vi "Read Return Address.vi"(11 "PreAddressedMsg in":refnum<class "PreAddressedMsg.lvclass">) -> (1 "Return Priority (Normal)":T1=enum."Normal", 2 "Return Address":refnum<class "Message Enqueuer.lvclass">)   [LabVIEW 2017, in "AbstractMessages.lvlib" / "PreAddressedMsg.lvclass"]
doc: "<License>\nCopyright © 2017 Composed Systems, LLC | All rights reserved\nwww.composed.io\n\nAuthor: Ethan Stern <ethan.stern@composed.io>\n\nThis software is provided \"AS IS\" WITHOUT WARRANTIES, either express or implied, AND IS FOR EDUCATIONAL PURPOSES ONLY.\n</License>"
uses:
  PreAddressedMsg.lvclass
  <vilib>/ActorFramework/Message Enqueuer/Message Enqueuer.lvclass
  <vilib>/ActorFramework/Message Enqueuer/Message Priority.ctl
  PreAddressedMsg.lvclass/PreAddressedMsg.ctl
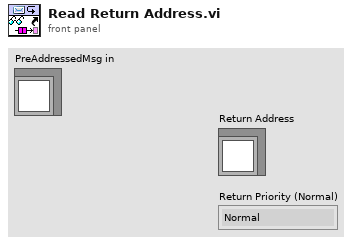
[diagram p1: front panel]
types:
  T1 = typedef "Actor Framework.lvlib/Message Enqueuer.lvclass/Message Priority.ctl" = enum16{"Low", "Normal", "High"}
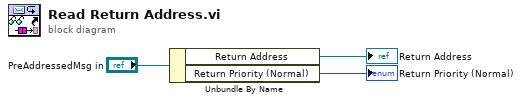
[diagram p0: block diagram]
diagram:
  n1 = Unbundle By Name("PreAddressedMsg in") -> ("Return Address"=→"Return Address":refnum<class "Message Enqueuer.lvclass">, "Return Priority (Normal)"=→"Return Priority (Normal)":T1)
